vi "console.vi"(8 "error in (no error)":errorcluster, 11 "console.provider in":refnum<class "console.provider.lvclass">) -> (0 "error out":errorcluster)   [LabVIEW 2021, in "console.provider.lvclass"]
uses:
  console.provider.lvclass
  console.provider.lvclass/console.provider.ctl
panel:
  in  "console":i32(listbox)
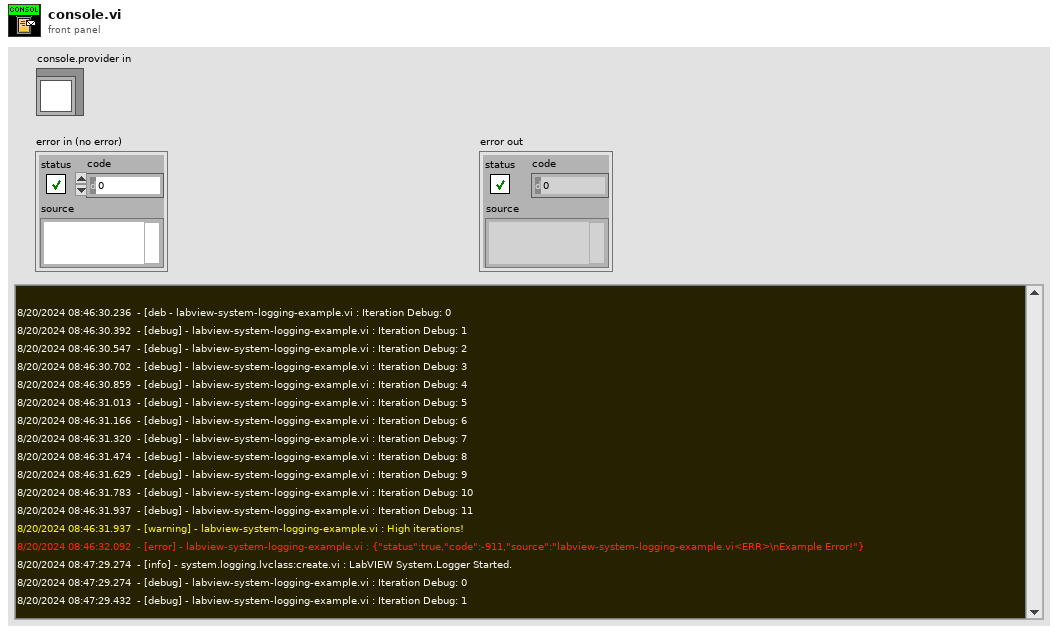
[diagram p1: front panel]
types:
  T1 = typedef "system.logging.lvclass/log_entry.ctl" = cluster{"severity":T2, "message":string, "origin":string, "datetime":timestamp}
  T2 = typedef "system.logging.lvclass/severity.ctl" = enum8{"trace", "debug", "info", "warning", "error"}
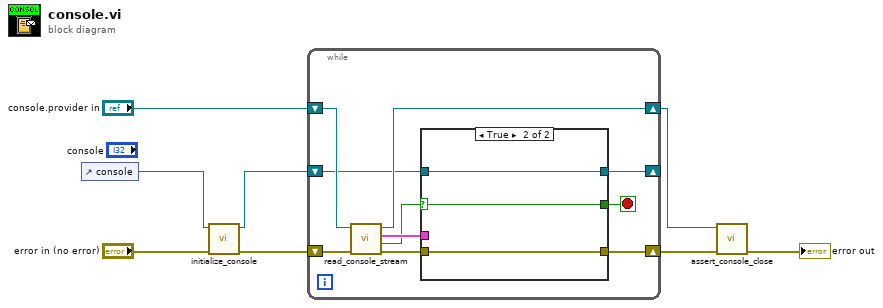
[diagram p0: block diagram]
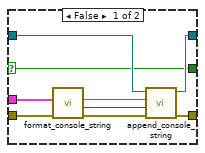
[diagram p2: hidden frame]
diagram:
  n1 = control-ref of="console"() -> (w5:refnum<vi>)
  n2 = call "initialize_console.vi"("error in (no error)"="error in (no error)", "console (in)"=w5) -> ("error out"=w6:errorcluster, "reference out"=w4:refnum<vi>)  [unwired: 8 in]
  n3 = while {
    shift-right: [w15] -> w3
    shift-left: w6 -> [w18]
    shift-right: [w16] -> w2
    shift-left: "console.provider in" -> [w17]
    shift-right: [w13] -> _
    shift-left: w4 -> [w14]
    stop <- w9 stop-if-true
    n4 = call "read_console_stream.vi"("error in (no error)"=w18, "console.provider in"=w17) -> ("error out"=w12:errorcluster, "abort"=w10:bool, "log"=w11:T1, "console.provider out"=w16:refnum<class "console.provider.lvclass">)  [unwired: 6 in]
    n5 = case shown="True" w10 {
      selector: w10 -> [w19 w28]
      tunnel: [w27 w29] -> w15
      tunnel: w14 -> [w26 w30]
      tunnel: [w25 w30] -> w13
      tunnel: w12 -> [w21 w29]
      tunnel: w11 -> [w20 _]
      tunnel: [w19 w28] -> w9
      frame False {
        n6 = call "format_console_string.vi"("error in (no error)"=w21, "log entry"=w20) -> ("error out"=w24:errorcluster, "color"=w22:u32, "text"=w23:string)  [unwired: 7 in]
        n7 = call "append_console_string.vi"("error in (no error)"=w24, "color"=w22, "newline"=w23, "console (in)"=w26) -> ("error out"=w27:errorcluster, "reference out"=w25:refnum<vi>)  [unwired: 6 in]
      }
      frame True {
      }
    }
  }
  n8 = call "assert_console_close.vi"("error in (no error)"=w3, "console.provider in"=w2) -> ("error out"=→"error out":errorcluster)  [unwired: 9 in]
